vi "Read Value.vi"(8 "error in":errorcluster, 11 "PowerSupply MSG in":refnum<class "PowerSupply MSG.lvclass">) -> (0 "error out":errorcluster, 2 "val":u8, 3 "PowerSupply MSG out":refnum<class "PowerSupply MSG.lvclass">)   [LabVIEW 2014, in "Controller.lvlib" / "PowerSupply MSG.lvclass"]
uses:
  PowerSupply MSG.lvclass
  PowerSupply MSG.lvclass/PowerSupply MSG.ctl
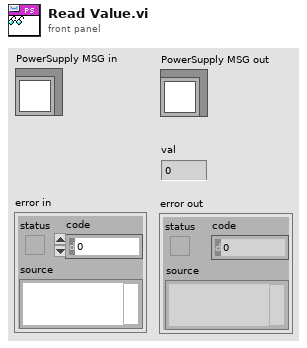
[diagram p1: front panel]
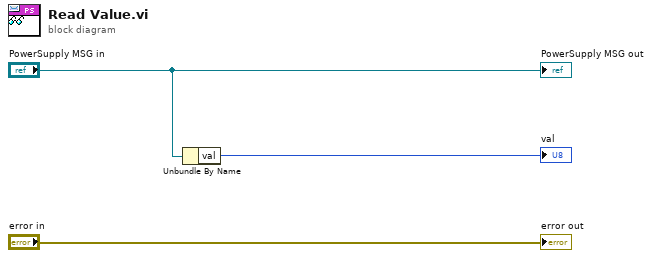
[diagram p0: block diagram]
diagram:
  n1 = Unbundle By Name("PowerSupply MSG in") -> ("val"=→"val":u8)
  "error out" <- "error in"
  "PowerSupply MSG out" <- "PowerSupply MSG in"
